vi "Run.vi"(8 "error in (no error)":errorcluster, 9 "s on last turn":dbl, 10 "Maze (0: Empty, -1: Enemy. >0: Teammate":i32[][](array[numeric]), 11 "Scout In":refnum<class "Scout.lvclass">) -> (0 "error out":errorcluster, 1 "Direction":T1, 2 "Action":T2, 3 "Scout Out":refnum<class "Scout.lvclass">, 4 "Replicated":refnum<class "Square.lvclass">)   [LabVIEW 2015, in "Scout.lvclass"]
uses:
  Scout.lvclass
  Type Defs/Action Enum.ctl
  Type Defs/Direction Enum.ctl
  Square/Square.lvclass
  Formics/Attack Options.ctl
  Scout.lvclass/Scout.ctl
  Formics/Formics.lvclass
  Type Defs/SB Type Defs.lvlib
panel:
  in  "Status":string
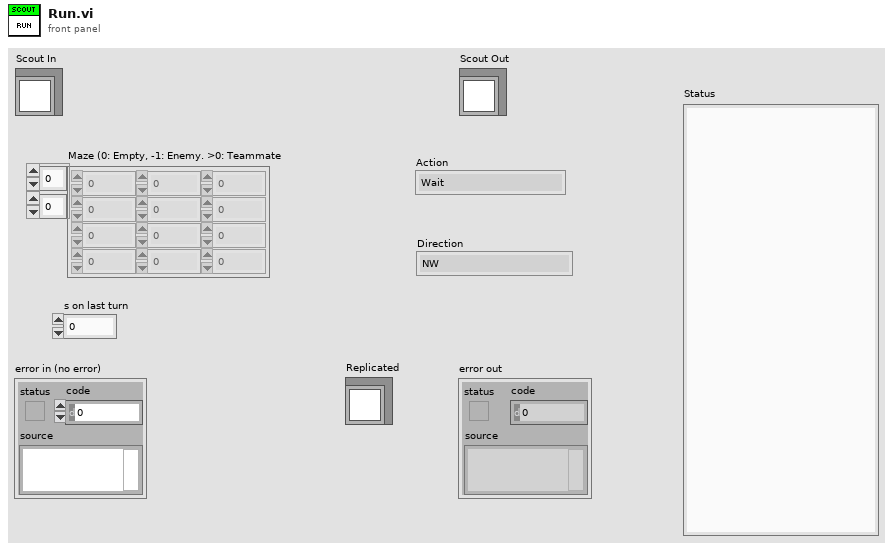
[diagram p1: front panel]
types:
  T1 = typedef "SB Type Defs.lvlib/Direction Enum.ctl" = enum16{"NW", "N", "NE", "E", "SE", "S", "SW", "W"}
  T2 = typedef "SB Type Defs.lvlib/Action Enum.ctl" = enum16{"Wait", "Move", "Attack", "Replicate"}
  T3 = typedef "Formics.lvclass/Attack Options.ctl" = enum16{"Attack", "Run", "Distract"}
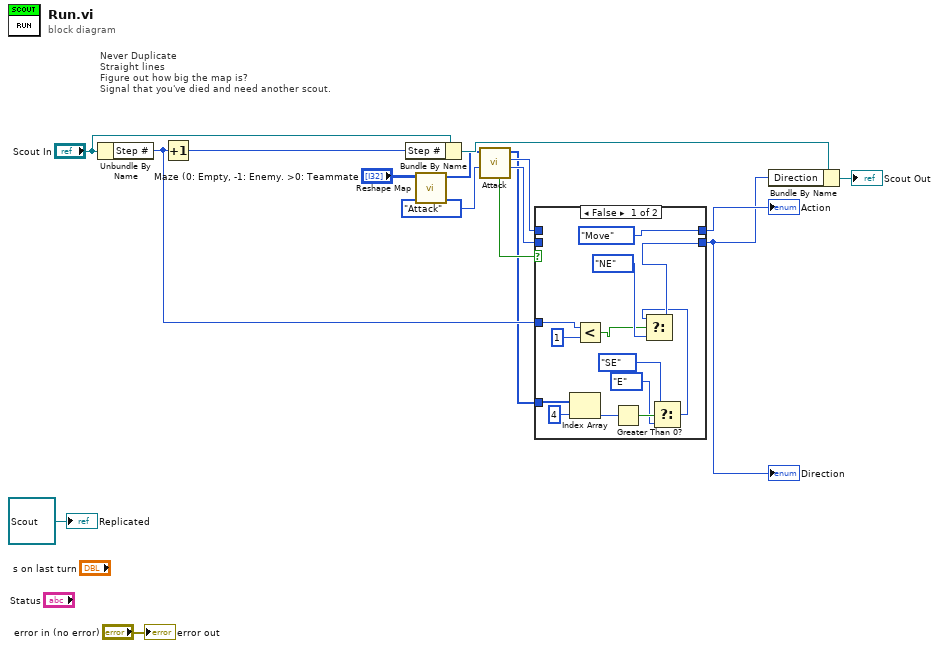
[diagram p0: block diagram]
diagram:
  # "Never Duplicate\nStraight lines\nFigure out how big the map is?\nSignal that you've died and need another scout."
  n1 = Unbundle By Name("Scout In") -> ("Step #"=w4:i32)
  n2 = Increment(x=w4) -> (x+1=w13:i32)
  n3 = Bundle By Name(cluster="Scout In", "Step #"=w13) -> (w3:refnum<class "Scout.lvclass">)
  n4 = call "Reshape Map.vi"("Maze (0: Empty, -1: Enemy. >0: Teammate"="Maze (0: Empty, -1: Enemy. >0: Teammate") -> ("Map"=w2:i32[])  [unwired: 9 in, 1 out]
  n5 = call "Attack.vi"("Attack?"=Attack_Options."Attack", "Maze (0: Empty, -1: Enemy. >0: Teammate"=w2) -> ("Direction"=w6:i32, "Action"=w8:T2, "Maze (0: Empty, -1: Enemy. >0: Teammate 2"=w1:i32[], "Enemy Found?"=w9:bool)  [unwired: 4 in, 2 out]
  n6 = case shown="False" w9 {
    tunnel: w8 -> [_ w30]
    tunnel: [Action_Enum."Move" ("Action") w30] -> w7
    tunnel: w6 -> [_ w31]
    tunnel: [w25 w31] -> w5
    tunnel: w4 -> [w27 _]
    tunnel: w1 -> [w23 _]
    frame False {
      n7 = Index Array(array=w23, index=4) -> (element=w21:i32)
      n8 = Less?(x=w27, y=1) -> (x < y?=w24:bool)
      n9 = Greater Than 0?(x=w21) -> (x > 0?=w20:bool)
      n10 = Select(t=Direction_Enum."SE", s=w20, f=Direction_Enum."E" ("t")) -> (s? t:f=w17:T1)
      n11 = Select(t=w17, s=w24, f=Direction_Enum."NE" ("Direction")) -> (s? t:f=w25:T1)
    }
    frame True {
    }
  }
  "Action" <- w7
  "Direction" <- w5
  n12 = Bundle By Name(cluster=w3, "Direction"=w5) -> (→"Scout Out":refnum<class "Scout.lvclass">)
  "error out" <- "error in (no error)"
  "Replicated" <- refnum<class "Scout.lvclass"> refnum ("Replicated")
